vi "controlador_motor_dc.vi"() -> ()   [LabVIEW 2025]
panel:
  in  "Desfase ref":dbl(slide) scale=0.0..2.0
  out "V Motor":dbl(slide) scale=0.0..5500.0
  in  "Boolean":bool caption="Limpiar XY Graph"
  out "rpm":dbl
  out "V":dbl
  in  "SP Modo Manual":dbl(slide) scale=0.0..5.0
  out "REVS":dbl caption="rpm"
  out "Modo actual":string
  in  "stop":bool
  in  "Selector de modo":u16(ring) items=["Manual", "Control Integral", "Seguidor Cuadrada", "Seguidor Triangular"]
  in  "SP Control Integral":dbl(slide) scale=0.0..5500.0
  out "count":dbl
  out "GRAPH 2":dynamicdata(graph)
  out "XY Graph":cluster{dbl[], dbl[]}(graph)
  out "GRAPH":dynamicdata(graph)
  out "v":dbl
  out "u":dbl
  out "x2":dbl
  out "x1":dbl
  # "CONTROL DE VELOCIDAD MOTOR"
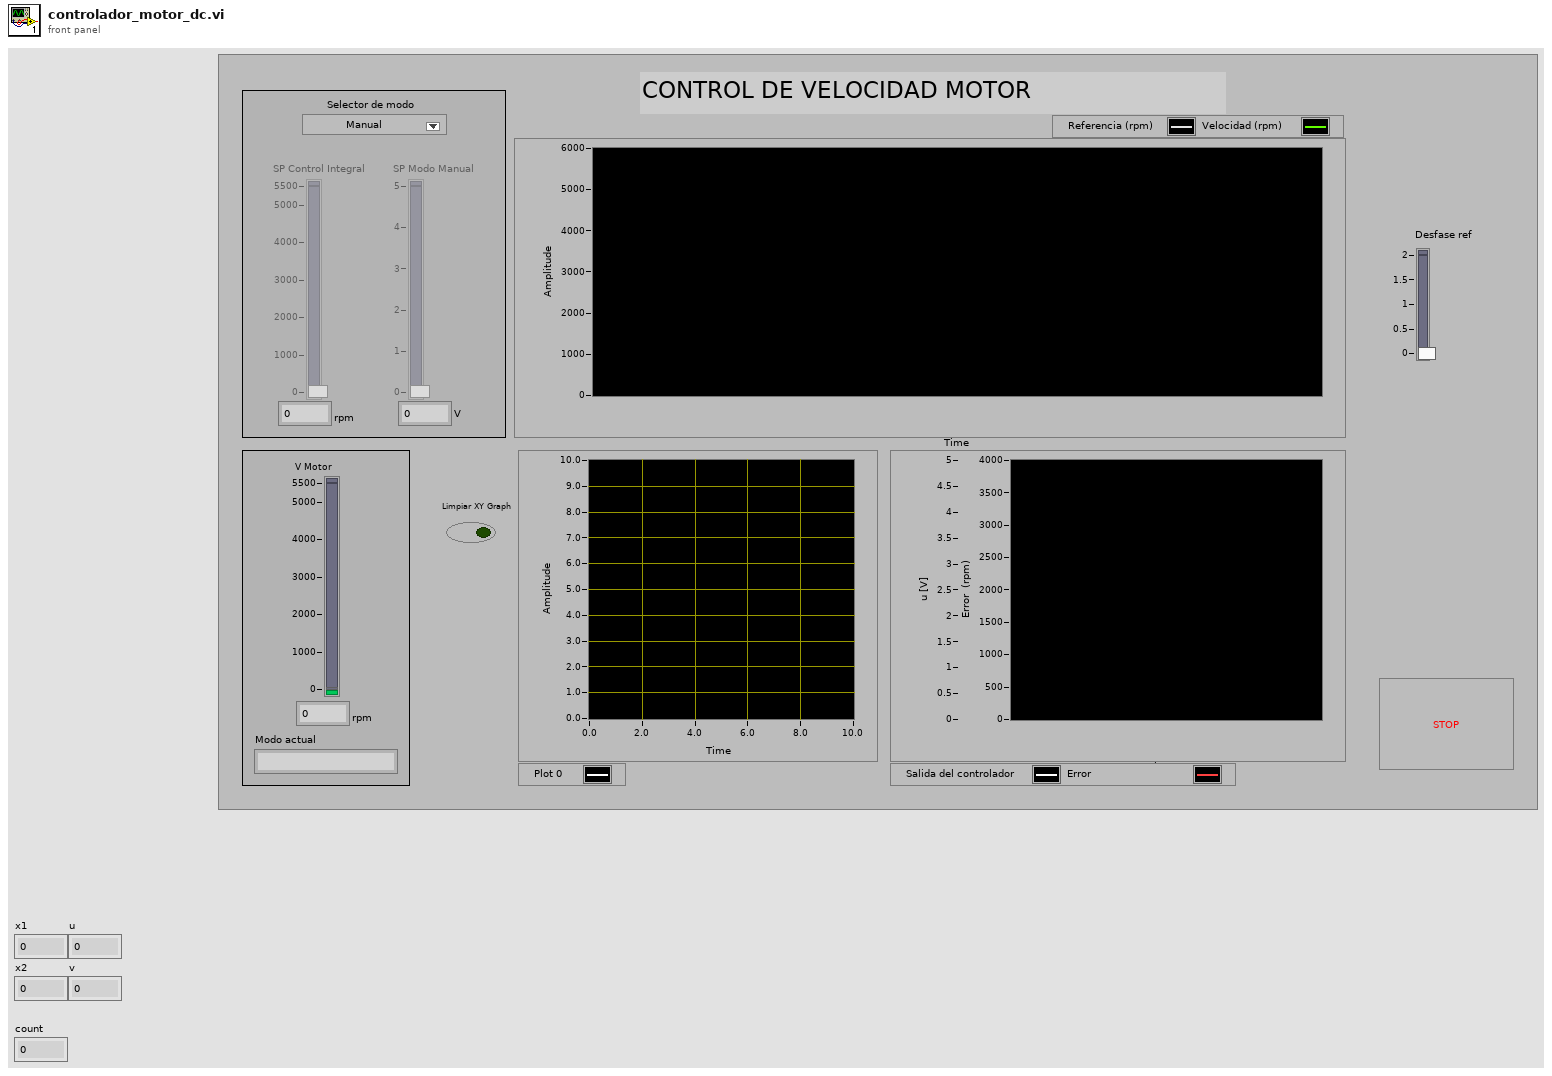
[diagram p1: front panel]
types:
  T1 = enum8{"Enabled", "Disabled", "Disabled and Grayed Out"}
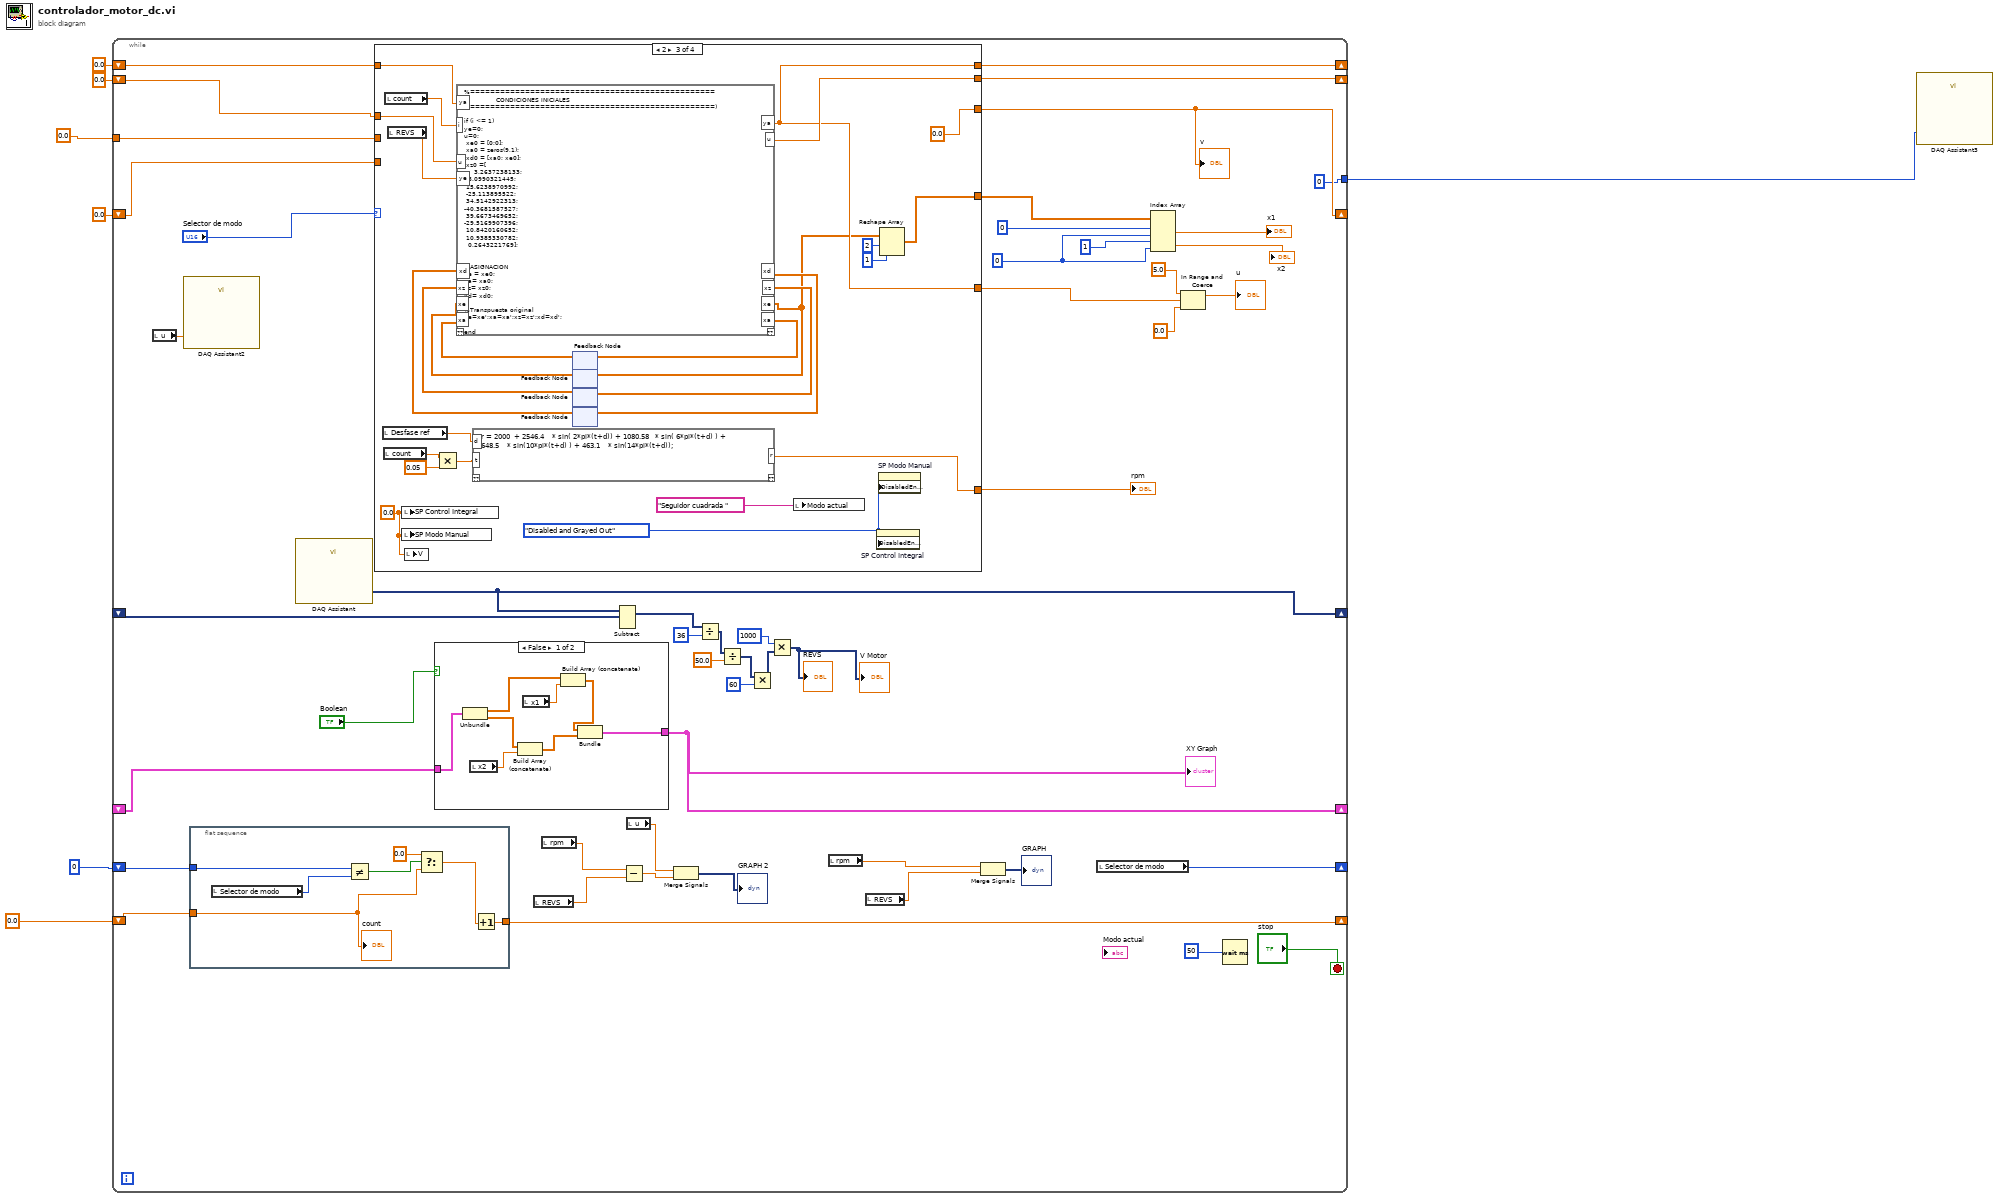
[diagram p0: block diagram]
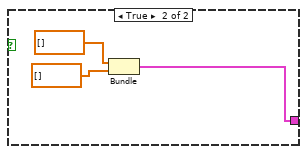
[diagram p2: hidden frame]
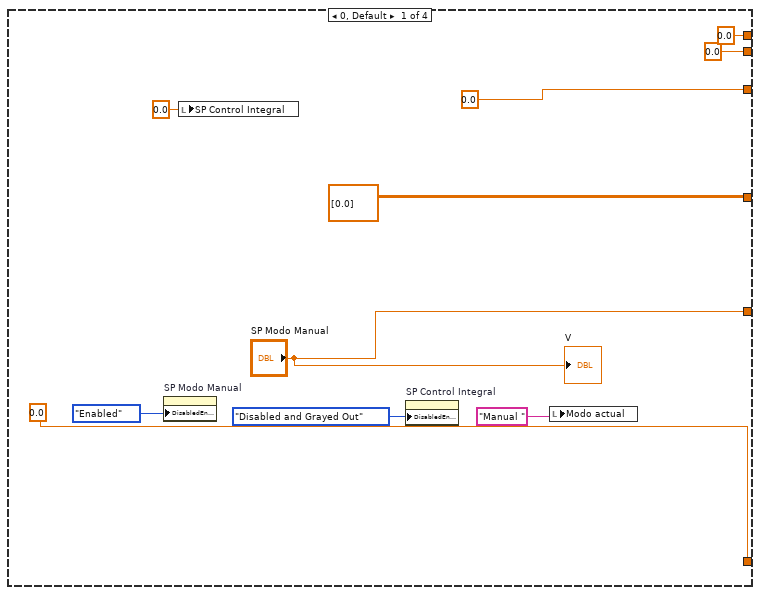
[diagram p3: hidden frame]
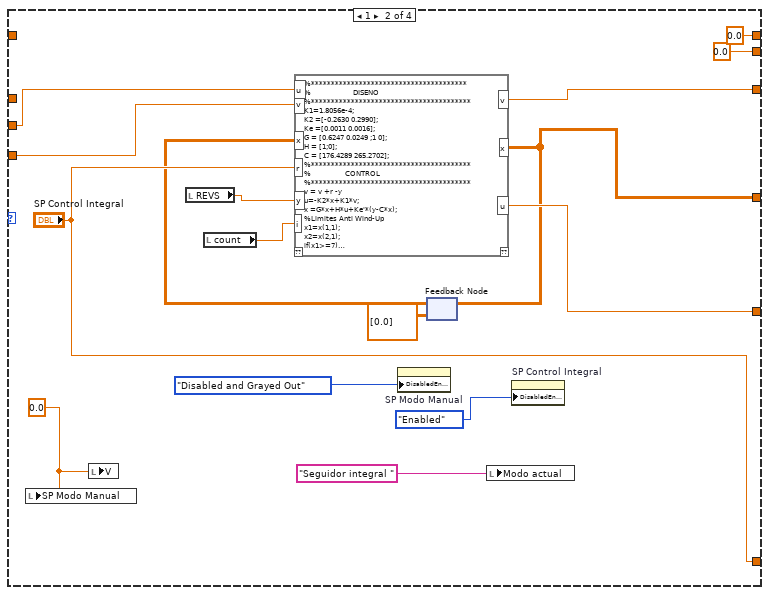
[diagram p4: hidden frame]
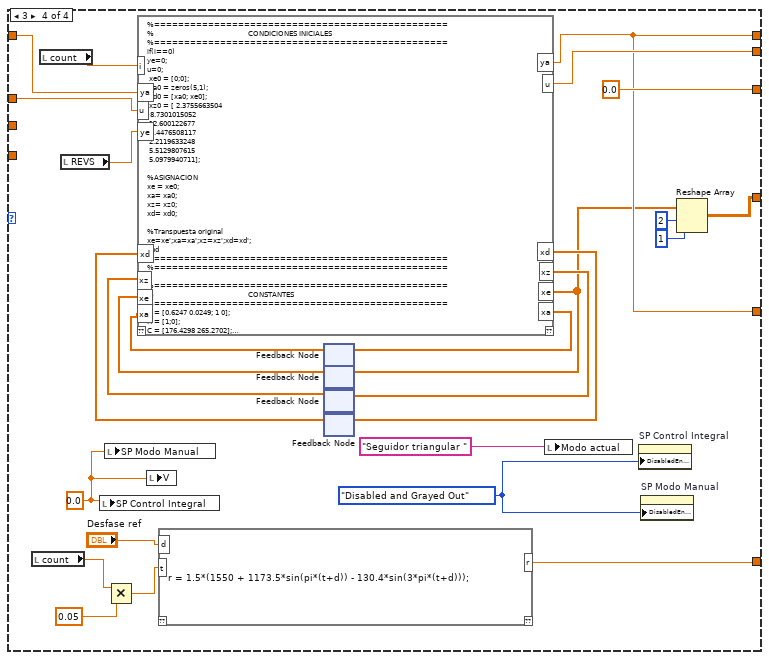
[diagram p5: hidden frame]
diagram:
  n1 = while {
    shift-right: [w44] -> _
    shift-left: 0.0 -> [w46]
    tunnel: [0] -> w7
    shift-right: [w33] -> _
    shift-left: _ -> [w35]
    shift-right: [w27] -> _
    shift-left: _ -> [w28]
    shift-right: [w20] -> _
    shift-left: 0 -> [w21]
    shift-right: [w19] -> _
    shift-left: 0.0 -> [w18]
    shift-right: [w13] -> _
    shift-left: 0.0 -> [w12]
    shift-right: [w11] -> _
    shift-left: 0.0 -> [w10]
    tunnel: 0.0 -> [w8]
    stop <- "stop" stop-if-true
    w50 = 0
    n2 = local read "u"() -> (w43:dbl)
    n3 = call "DAQ Assistant2"("data"=w43) -> ()  [unwired: 17 in, 2 out]
    n4 = flat-sequence {
      tunnel: w21 -> [w63]
      tunnel: [w58] -> w19
      tunnel: w18 -> [w57]
      frame #0 {
        n5 = local read "Selector de modo"() -> (w62:u16)
        n6 = Not Equal?(x=w63, y=w62) -> (x != y?=w61:bool)
        n7 = Select(t=0.0, s=w61, f=w57) -> (s? t:f=w59:dbl)
        n8 = Increment(x=w59) -> (x+1=w58:dbl)
        "count" <- w57
      }
    }
    n9 = call "DAQ Assistant"() -> ("data"=w33:dynamicdata)  [unwired: 16 in, 3 out]
    n10 = case shown="2" "Selector de modo" {
      tunnel: ["SP Modo Manual" w99 w119 w138] -> w9
      tunnel: [dbl[][] [[0.0]] w92 w109 w133] -> w45
      tunnel: [0.0 w98 0.0 0.0] -> w44
      tunnel: w46 -> [_ w97 _ _]
      tunnel: [0.0 ("Scalar") "SP Control Integral" w104 w131] -> w26
      tunnel: [0.0 0.0 w119 w138] -> w13
      tunnel: w12 -> [_ _ w107 w141]
      tunnel: [0.0 0.0 w120 w140] -> w11
      tunnel: w10 -> [_ _ w106 w139]
      tunnel: w8 -> [_ w86 _ _]
      frame 0, Default {
        n11 = property on="SP Modo Manual" class="Slide (strict)"("DisabledEnum"=T1."Enabled" ("Disabled")) -> ()  [unwired: 2 in, 2 out]
        n12 = local write "SP Control Integral"(0.0 ("SP Control Integral")) -> ()
        n13 = property on="SP Control Integral" class="Slide (strict)"("DisabledEnum"=T1."Disabled and Grayed Out" ("Disabled")) -> ()  [unwired: 2 in, 2 out]
        n14 = local write "Modo actual"("Manual ") -> ()
        "V" <- "SP Modo Manual"
      }
      frame 1 {
        w87 = 0.0
        n15 = local write "SP Modo Manual"(w87) -> ()
        n16 = local write "V"(w87) -> ()
        n17 = local read "REVS"() -> (w96:dbl)
        n18 = local read "count"() -> (w94:dbl)
        n19 = property on="SP Modo Manual" class="Slide (strict)"("DisabledEnum"=T1."Disabled and Grayed Out" ("Disabled")) -> ()  [unwired: 2 in, 2 out]
        n20 = feedback #1(dbl[][] [[0.0]]) -> (w93:dbl[][])
        n21 = script code="%***************************************\n%                     DISENO\n%****************************************\nK1=1.8056e-4;\nK2 =[-0.2630 0.2990];\nKe =[0.0011 0.0016];\nG = [0.6247 0.0249 ;1 0];\nH = [1;0];\nC = [176.4289 265.2702];\n%****************************************\n%                 CONTROL\n%****************************************\nv = v +r -y\nu=-K2*x+K1*v;\nx =G*x+H*u+Ke'*(y-C*x);\n%Limites Anti Wind-Up\nx1=x(1,1);\nx2=x(2,1);\nif(x1>=7)\nx1=7;\nend\nif(x2>=7)\nx2=7;\nend\nif (u>=5)\nu=5;\nend\nx =[x1;x2];\nif(v>30e3)\nv = 30e3;\nend\nif(v<1713.45)\nv=1713.45;\nend"("v"=w97, "r"="SP Control Integral", "y"=w96, "x"=w93, "i"=w94, "u"=w86) -> ("v"=w98:dbl, "u"=w99:dbl, "x"=w92:dbl[][])  [unwired: 1 in, 1 out]
        n22 = feedback-in #1(w92) -> ()
        n23 = local write "Modo actual"("Seguidor integral ") -> ()
        n24 = property on="SP Control Integral" class="Slide (strict)"("DisabledEnum"=T1."Enabled" ("Disabled")) -> ()  [unwired: 2 in, 2 out]
      }
      frame 2 {
        w123 = 0.0 ("SP Control Integral")
        w124 = T1."Disabled and Grayed Out" ("Disabled")
        n25 = local read "Desfase ref"() -> (w105:dbl)
        n26 = local read "count"() -> (w101:dbl)
        n27 = local read "count"() -> (w122:dbl)
        n28 = local read "REVS"() -> (w121:dbl)
        n29 = local write "SP Control Integral"(w123) -> ()
        n30 = local write "SP Modo Manual"(w123) -> ()
        n31 = local write "V"(w123) -> ()
        n32 = Multiply(x=w101, y=0.05) -> (x*y=w102:dbl)
        n33 = script code="r = 2000  + 2546.4    * sin( 2*pi*(t+d)) + 1080.58   * sin( 6*pi*(t+d) ) + 648.5    * sin(10*pi*(t+d) ) + 463.1    * sin(14*pi*(t+d));"("t"=w102, "d"=w105) -> ("r"=w104:dbl)  [unwired: 1 in, 1 out]
        n34 = feedback #2() -> (w115:dbl[])  [unwired: 1 in]
        n35 = feedback #3() -> (w114:dbl[])  [unwired: 1 in]
        n36 = feedback #4() -> (w113:dbl[])  [unwired: 1 in]
        n37 = feedback #5() -> (w112:dbl[])  [unwired: 1 in]
        n38 = script code="%=================================================\n%             CONDICIONES INICIALES\n%=================================================)\n\nif (i <= 1)\nye=0;\nu=0;\n xe0 = [0;0];\n xa0 = zeros(9,1);\n xd0 = [xa0; xe0];\n xz0 =[\n     3.2637238133;\n -8.0990321445;\n 15.6238970992;\n -25.113895522;\n 34.5142922313;\n-40.3681587527;\n 39.6673469652;\n-29.5169907396;\n 10.8420160652;\n 10.9385330782;\n  0.2643221769];\n\n\n%ASIGNACION\nxe = xe0;                            \nxa= xa0;\nxz= xz0;                            \nxd= xd0;\n\n%Transpuesta original\nxe=xe';xa=xa';xz=xz';xd=xd';\n\nend\n\n\n\n\n\n\n%=================================================\n%=================================================\n\n%=================================================\n%                                               CONSTANTES\n%=================================================\nG = [0.6247 0.0249; 1 0];\nH = [1;0];\nC = [176.4298 265.2702];\n\n\nKe =[0.001084215769946   0.001594163174481];\n\nke_a = [0.034548388316391  -0.044350564510259   0.056987975163788  -0.063136924258813   0.063137368102525  -0.056957140810380   0.045201464494327  -0.029021129725830   0.009999999970072];\n\nE =[1.000000000000745\n  -0.000000000033307\n   0.000000001000482\n  -0.000000027200529\n   0.000000725733218\n  -0.000020363852518\n   0.000148842645721\n  -0.028054767075925\n   0.228525474023322\n   0.635523128733625\n   0.329600781794658 ];\n\nAa = [2.902113032590308   1.000000000000000                   0                   0                   0                   0                   0                   0                   0;\n  -4.520147021340203                   0   1.000000000000000                   0                   0                   0                   0                   0                   0;\n   5.695717525925152                   0                   0   1.000000000000000                   0                   0                   0                   0                   0;\n  -6.313751514675045                   0                   0                   0   1.000000000000000                   0                   0                   0                   0;\n   6.313751514675045                   0                   0                   0                   0   1.000000000000000                   0                   0                   0;\n  -5.695717525925152                   0                   0                   0                   0                   0   1.000000000000000                   0                   0;\n   4.520147021340201                   0                   0                   0                   0                   0                   0   1.000000000000000                   0;\n  -2.902113032590308                   0                   0                   0                   0                   0                   0                   0   1.000000000000000;\n   1.000000000000000                   0                   0                   0                   0                   0                   0                   0                   0]\n\nBa =[  2.902113032590308;\n  -4.520147021340203;\n   5.695717525925152;\n  -6.313751514675045;\n   6.313751514675045;\n  -5.695717525925152;\n   4.520147021340201;\n  -2.902113032590308;\n   1.000000000000000];\n\nCa = [1     0     0     0     0     0     0     0     0];\nDa = 1;\nm = size(Aa,1);   \nAd = [Aa, zeros(m, 2); H*Ca, G];\ndisp(\"etapa1\")\n%=================================================\n%=================================================\n\n%=================================================\n%                                    TRANSPUESTAS REQUERIDAS\n%=================================================\nxe=xe';xa=xa';xz=xz';xd=xd';\n%=================================================\n%=================================================\n\n%=================================================\n%                                            CONTROL\n%=================================================\nxd = [ xa;xe ];\nxz = Ad * xz;\nu = E' * ( xz-xd );\nya = Ca * xa + Da * u;\nxe = G* xe + H * ya + Ke'*( ye - C*xe );\nxa = Aa * xa+ Ba * u + ke_a'*(ya - Ca*xa);\n%ye = C*xe;\n\nxe=xe';xa=xa';xz=xz';xd=xd';"("i"=w122, "ya"=w107, "u"=w106, "xd"=w112, "xz"=w113, "xe"=w114, "xa"=w115, "ye"=w121) -> ("xd"=w118:dbl[], "xz"=w117:dbl[], "xe"=w108:dbl[], "xa"=w116:dbl[], "ya"=w119:dbl, "u"=w120:dbl)  [unwired: 1 in, 1 out]
        n39 = feedback-in #2(w116) -> ()
        n40 = feedback-in #3(w108) -> ()
        n41 = feedback-in #4(w117) -> ()
        n42 = feedback-in #5(w118) -> ()
        n43 = local write "Modo actual"("Seguidor cuadrada ") -> ()
        n44 = property on="SP Control Integral" class="Slide (strict)"("DisabledEnum"=w124) -> ()  [unwired: 2 in, 2 out]
        n45 = property on="SP Modo Manual" class="Slide (strict)"("DisabledEnum"=w124) -> ()  [unwired: 2 in, 2 out]
        n46 = Reshape Array(w108, 2 ("dimension size"), 1 ("dimension size")) -> (w109:dbl[][])
      }
      frame 3 {
        w132 = 0.0 ("SP Control Integral")
        w150 = T1."Disabled and Grayed Out" ("Disabled")
        n47 = local read "count"() -> (w128:dbl)
        n48 = local read "count"() -> (w142:dbl)
        n49 = local read "REVS"() -> (w137:dbl)
        n50 = local write "SP Control Integral"(w132) -> ()
        n51 = local write "SP Modo Manual"(w132) -> ()
        n52 = Multiply(x=w128, y=0.05) -> (x*y=w129:dbl)
        n53 = local write "V"(w132) -> ()
        n54 = script code="r = 1.5*(1550 + 1173.5*sin(pi*(t+d)) - 130.4*sin(3*pi*(t+d)));"("t"=w129, "d"="Desfase ref") -> ("r"=w131:dbl)  [unwired: 1 in, 1 out]
        n55 = feedback #6() -> (w149:dbl[])  [unwired: 1 in]
        n56 = feedback #7() -> (w148:dbl[])  [unwired: 1 in]
        n57 = feedback #8() -> (w146:dbl[])  [unwired: 1 in]
        n58 = feedback #9() -> (w144:dbl[])  [unwired: 1 in]
        n59 = script code="%=================================================\n%                                               CONDICIONES INICIALES\n%=================================================\nif(i==0)\nye=0;\nu=0;\n xe0 = [0;0];\n xa0 = zeros(5,1);\n xd0 = [xa0; xe0];\n xz0 = [ 2.3755663504\n-8.7301015052\n 12.600122677\n-8.4476508117\n 2.2119633248\n 5.5129807615\n 5.0979940711];\n\n%ASIGNACION\nxe = xe0;                            \nxa= xa0;\nxz= xz0;                            \nxd= xd0;\n\n%Transpuesta original\nxe=xe';xa=xa';xz=xz';xd=xd';\nend\n%=================================================\n%=================================================\n\n%=================================================\n%                                               CONSTANTES\n%=================================================\nG = [0.6247 0.0249; 1 0];\nH = [1;0];\nC = [176.4298 265.2702];\n\nKe = [ 0.001084215769946   0.001594163174481];\nke_a = [0.099369754013524  -0.185422789507507   0.185537651884478  -0.095145289849285   0.019999783164454];\n\nE=[ 1.000000000000000\n   0.000000000000054\n  -0.000000000000846\n  -0.000000061371594\n   0.000073888728845\n   0.633951587678753\n   0.024968584281983];\n\nAa = [\n   4.757389729567011   1.000000000000000                   0                   0                   0;\n  -9.277536750907213                   0   1.000000000000000                   0                   0;\n   9.277536750907213                   0                   0   1.000000000000000                   0;\n  -4.757389729567012                   0                   0                   0   1.000000000000000;\n   1.000000000000000                   0                   0                   0                   0];\n\nBa =[4.757389729567011;\n  -9.277536750907213;\n   9.277536750907213;\n  -4.757389729567012;\n   1.000000000000000];\n\nCa = [1 0 0 0 0];\nDa = 1;\nm = size(Aa,1);   \nAd = [Aa, zeros(m, 2); H*Ca, G];\n%=================================================\n%=================================================\n\n%=================================================\n%                                    TRANSPUESTAS REQUERIDAS\n%=================================================\nxe=xe';xa=xa';xz=xz';xd=xd';\n%=================================================\n%=================================================\n\n%=================================================\n%                                            CONTROL\n%=================================================\nxd = [ xa;xe ];\nxz = Ad * xz;\nu = E' * ( xz-xd );\nya = Ca * xa + Da * u;\nxe = G* xe + H * ya + Ke'*( ye - C*xe );\nxa = Aa * xa+ Ba * u + ke_a'*(ya - Ca*xa);\n%ye = C*xe;\n\nxe=xe';xa=xa';xz=xz';xd=xd';"("i"=w142, "ya"=w141, "u"=w139, "xd"=w144, "xz"=w146, "xe"=w148, "xa"=w149, "ye"=w137) -> ("xd"=w145:dbl[], "xz"=w147:dbl[], "xe"=w136:dbl[], "xa"=w143:dbl[], "ya"=w138:dbl, "u"=w140:dbl)  [unwired: 1 in, 1 out]
        n60 = feedback-in #6(w143) -> ()
        n61 = feedback-in #7(w136) -> ()
        n62 = feedback-in #8(w147) -> ()
        n63 = feedback-in #9(w145) -> ()
        n64 = local write "Modo actual"("Seguidor triangular ") -> ()
        n65 = property on="SP Control Integral" class="Slide (strict)"("DisabledEnum"=w150) -> ()  [unwired: 2 in, 2 out]
        n66 = property on="SP Modo Manual" class="Slide (strict)"("DisabledEnum"=w150) -> ()  [unwired: 2 in, 2 out]
        n67 = Reshape Array(w136, 2 ("dimension size"), 1 ("dimension size")) -> (w133:dbl[][])
      }
    }
    "v" <- w44
    "rpm" <- w26
    n68 = case shown="False" "Boolean" {
      tunnel: w28 -> [w71 _]
      tunnel: [w64 w72] -> w27
      frame False {
        n69 = Unbundle(w71) -> (w70:dbl[], w69:dbl[])
        n70 = local read "x2"() -> (w67:dbl)
        n71 = Build Array (concatenate)(w69, w67) -> (w66:dbl[])
        n72 = local read "x1"() -> (w68:dbl)
        n73 = Build Array (concatenate)(w70, w68) -> (w65:dbl[])
        n74 = Bundle(w65, w66) -> (w64:cluster{dbl[], dbl[]})  [unwired: 1 in]
      }
      frame True {
        n75 = Bundle(dbl[] [], dbl[] []) -> (w72:cluster{dbl[], dbl[]})  [unwired: 1 in]
      }
    }
    "XY Graph" <- w27
    n76 = local read "REVS"() -> (w24:dbl)
    n77 = local read "rpm"() -> (w25:dbl)
    n78 = Subtract(1:w35, 2:w33) -> (0:w34:dynamicdata)  [unwired: 1 in, 1 out]
    n79 = Subtract(x=w25, y=w24) -> (x-y=w23:dbl)
    n80 = local read "u"() -> (w22:dbl)
    n81 = Merge Signals(w22, w23) -> (→"GRAPH 2":dynamicdata)
    n82 = Divide(x=w34, y=36) -> (x/y=w38:dynamicdata)
    n83 = Divide(x=w38, y=50.0) -> (x/y=w39:dynamicdata)
    n84 = Multiply(x=w39, y=60) -> (x*y=w37:dynamicdata)
    n85 = Multiply(x=1000 ("y"), y=w37) -> (x*y=→"REVS" →"V Motor":dynamicdata)
    n86 = local read "rpm"() -> (w32:dbl)
    n87 = local read "REVS"() -> (w30:dbl)
    n88 = Merge Signals(w32, w30) -> (→"GRAPH":dynamicdata)
    n89 = local read "Selector de modo"() -> (w20:u16)
    n90 = Index Array(array=w45, index (row) #1=0, index (col) #1=w50, index (row) #2=1 ("disabled index (col)"), index (col) #2=w50) -> (element #1=→"x1":dbl, element #2=→"x2":dbl)
    n91 = In Range and Coerce(upper limit=5.0, x=w9, lower limit=0.0) -> (coerced(x)=→"u":dbl)  [unwired: 1 out]
    n92 = Wait (ms)(milliseconds to wait=50) -> ()  [unwired: 1 out]
  }
  n93 = call "DAQ Assistant3"("data"=w7) -> ()  [unwired: 17 in, 2 out]
